vi "ES Cycle Count.vi"(7 "SSG Average Total Active Power":dbl, 8 "Error In":errorcluster, 10 "ES String Data":T3, 11 "ES System Data":T1={"Voltage"=0.0, "Current"=0.0, "SOC Avg"=0.0, "Faults"=0, "Alarms"=0, "# Strings"=0, "Max Temp"=0, "Min Temp"=0, "Max Cell Voltage"=0.0, "Min Cell Voltage"=0.0, "Energy Capacity"=0.0, "Energy Remaining"=0.0, "SOC Min"=0.0, "SOC Max"=0.0, "ES Fault"=FALSE, "String Select"=enum."3 Strings", "ES Com Fault"=TRUE, "SOH Avg"=0.0}) -> (0 "error out":errorcluster, 1 "Write Data":string[](array[string]), 2 "Read Data":string[](array[string]), 3 "# cycles":dbl)   [LabVIEW 2014]
uses:
  Controls/ES String Array.ctl
  Controls/ES String Data.ctl
  Controls/ES System Data.ctl
  Controls/StringSelector.ctl
panel:
  out "Array":dbl[](array[numeric])
  out "# cycles per string":dbl
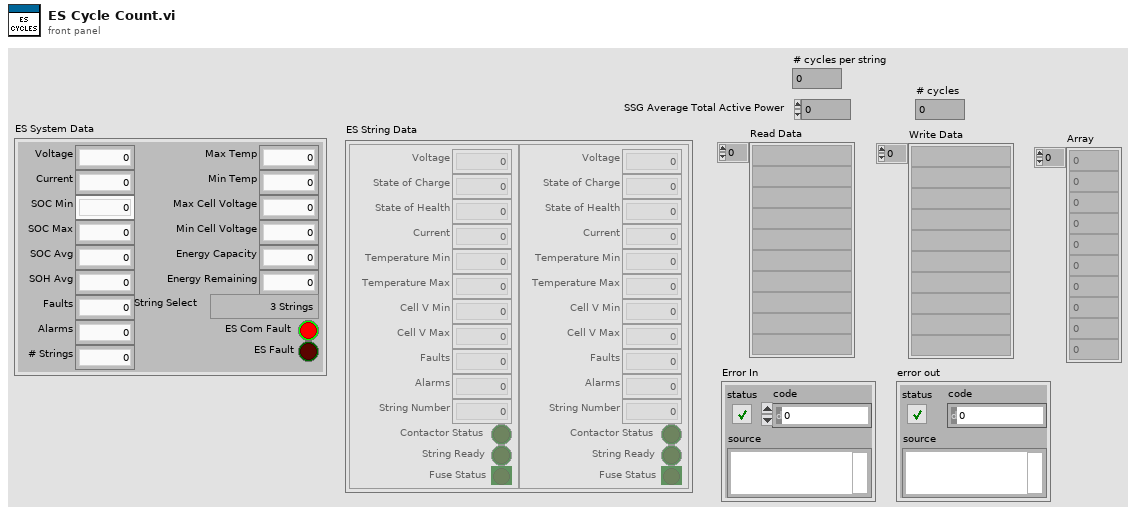
[diagram p1: front panel]
types:
  T1 = typedef "ES System Data.ctl" = cluster{"Voltage":sgl, "Current":sgl, "SOC Avg":sgl, "Faults":u16, "Alarms":u16, "# Strings":u16, "Max Temp":i16, "Min Temp":i16, "Max Cell Voltage":sgl, "Min Cell Voltage":sgl, "Energy Capacity":sgl, "Energy Remaining":sgl, "SOC Min":sgl, "SOC Max":sgl, "ES Fault":bool, "String Select":T2, "ES Com Fault":bool, "SOH Avg":sgl}
  T2 = typedef "StringSelector.ctl" = enum16{"1 String (1)", "1 String (2)", "1 String (3)", "2 Strings (1 2)", "2 Strings (2 3)", "2 Strings (1 3)", "3 Strings"}
  T3 = typedef "ES String Array.ctl" = T4[]
  T4 = typedef "ES String Data.ctl" = cluster{"Voltage":sgl, "State of Charge":sgl, "Current":sgl, "Temperature Min":i16, "Temperature Max":i16, "Faults":u16, "Alarms":u16, "String Number":u16, "Contactor Status":bool, "String Ready":bool, "Fuse Status":bool, "Cell V Max":dbl, "Cell V Min":dbl, "State of Health":sgl}
  T5 = enum16{"open", "replace", "create", "open or create", "replace or create", "replace or create with confirmation"}
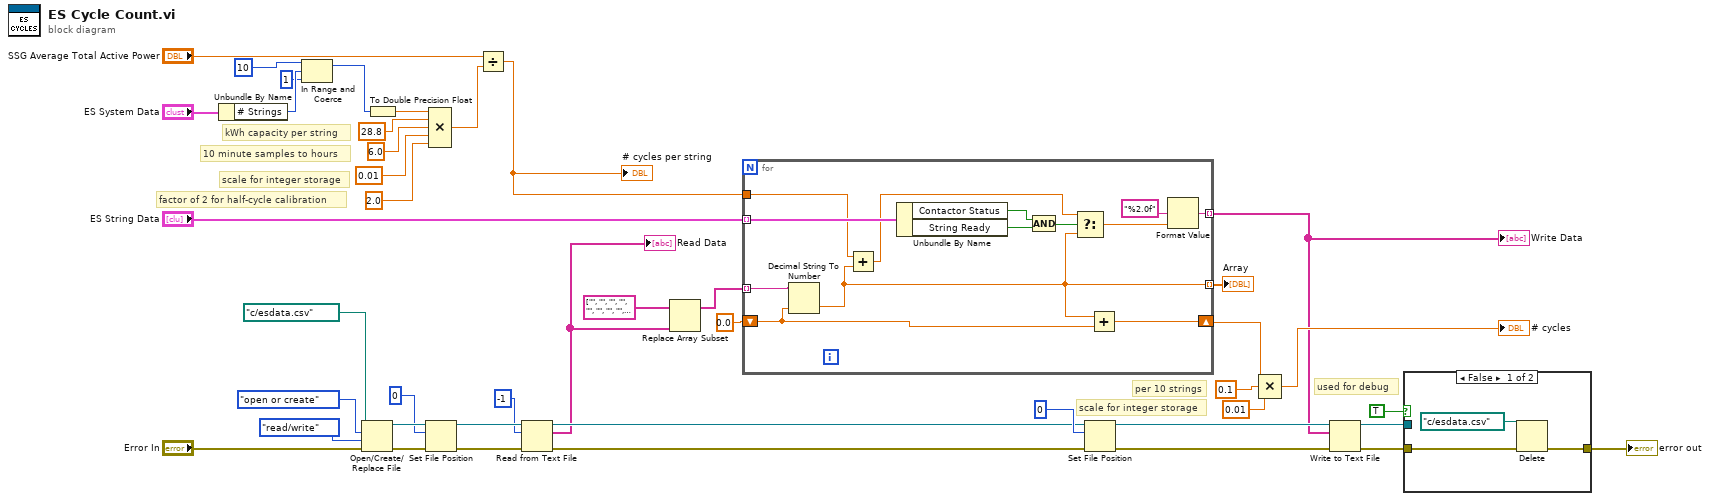
[diagram p0: block diagram]
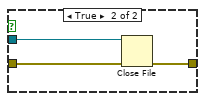
[diagram p2: hidden frame]
diagram:
  # "factor of 2 for half-cycle calibration"
  # "used for debug"
  # "scale for integer storage"
  # "per 10 strings"
  # "scale for integer storage"
  # "10 minute samples to hours"
  # "kWh capacity per string"
  n1 = Unbundle By Name("ES System Data") -> ("# Strings"=w9:u16)
  n2 = In Range and Coerce(upper limit=u16 10, x=w9, lower limit=u16 1) -> (coerced(x)=w8:u16)  [unwired: 1 out]
  n3 = Open/Create/Replace File(file path (use dialog)=path "c:/esdata.csv", error in="Error In", operation (0:open)=T5."open or create", access (0:read/write)=enum16{"read/write", "read-only", "write-only"}."read/write") -> (refnum out=w39:refnum<file>, error out=w40:errorcluster)  [unwired: 2 in, 1 out]
  n4 = To Double Precision Float(number=w8) -> (double precision float=w33:dbl)
  n5 = Set File Position(offset (in bytes) (0)=i64 0, refnum=w39, error in=w40) -> (refnum out=w35:refnum<file>, error out=w36:errorcluster)  [unwired: 1 in]
  n6 = Compound Arithmetic op=MULTIPLY(w33, 28.8 ("value"), 6.0 ("value"), 0.01 ("value"), 2.0 ("value")) -> (w30:dbl)
  n7 = Divide(x="SSG Average Total Active Power", y=w30) -> (x/y=w4:dbl)
  "# cycles per string" <- w4
  n8 = Read from Text File(file (use dialog)=w35, count=-1, error in=w36) -> (refnum out=w26:refnum<file>, text=w17:string[], error out=w27:errorcluster)  [unwired: 1 in, 1 out]
  "Read Data" <- w17
  n9 = Replace Array Subset(array=string[] ["", "", "", "", "", "", "", "", "", " "] ("Array"), new element=w17) -> (w16:string[])  [unwired: 1 in]
  n10 = for {
    tunnel: w4 -> [w48]
    tunnel: "ES String Data" -> [w56] mode=indexing
    tunnel: [w50] -> w3 mode=indexing
    shift-right: [w49] -> w13
    shift-left: 0.0 -> [w44]
    tunnel: w16 -> [w46] mode=indexing
    tunnel: [w45] -> w5 mode=indexing
    n11 = Decimal String To Number(string=w46, default (0L)=w44) -> (number=w45:dbl)  [unwired: 1 in, 1 out]
    n12 = Add(x=w48, y=w45) -> (x+y=w47:dbl)
    n13 = Unbundle By Name(w56) -> ("Contactor Status"=w55:bool, "String Ready"=w54:bool)
    n14 = Compound Arithmetic op=AND(w55, w54) -> (w53:bool)
    n15 = Select(t=w47, s=w53, f=w45) -> (s? t:f=w51:dbl)
    n16 = Add(x=w45, y=w44) -> (x+y=w49:dbl)
    n17 = Format Value(format string="%2.0f", value (0)=w51) -> (output string=w50:string)  [unwired: 1 in]
  }
  "Write Data" <- w3
  "Array" <- w5
  n18 = Set File Position(offset (in bytes) (0)=i64 0, refnum=w26, error in=w27) -> (refnum out=w24:refnum<file>, error out=w25:errorcluster)  [unwired: 1 in]
  n19 = Compound Arithmetic op=MULTIPLY(w13, 0.1 ("y"), 0.01 ("value")) -> (→"# cycles":dbl)
  n20 = Write to Text File(file (use dialog)=w24, text=w3, error in=w25) -> (refnum out=w21:refnum<file>, error out=w23:errorcluster)  [unwired: 1 in, 1 out]
  n21 = case shown="False" TRUE {
    tunnel: w23 -> [w59 w62]
    tunnel: [w58 w61] -> w22
    tunnel: w21 -> [_ w60]
    frame False {
      n22 = Delete(path (use dialog)=path "c:/esdata.csv" ("file path (use dialog)"), error in=w59) -> (error out=w58:errorcluster)  [unwired: 3 in, 2 out]
    }
    frame True {
      n23 = Close File(refnum=w60, error in=w62) -> (error out=w61:errorcluster)  [unwired: 1 out]
    }
  }
  "error out" <- w22
